vi "Evaluate Calibration.vi"(6 "Calibration Type":string, 7 "Position":u32, 8 "Error in":errorcluster caption="Error in (no error)", 9 "DSPic Measurement":dbl, 10 "Actual Measurement":dbl, 11 "Calibration in":refnum<class "Calibration.lvclass">) -> (0 "Error out":errorcluster, 3 "Passed":bool)   [LabVIEW 2015, in "Calibration.lvclass"]
uses:
  Calibration.lvclass
  <vilib>/Cree, Inc/Cree Test Framework/Core Launcher/Core Manager Methods -- Enum.ctl
  CBTF Applications/Driver Board Testing/Main/Application/Application/Class/Driver Board Test.lvclass
  <vilib>/Cree, Inc/Cree Test Framework/Core Launcher/Core Launcher.lvlib
  <vilib>/Cree, Inc/Cree Test Framework/Classes/Data/Data Repo/Class/Data Repo.lvclass
  Test Class/Test Class.lvclass
  Classes/Application/Class/Application.lvclass
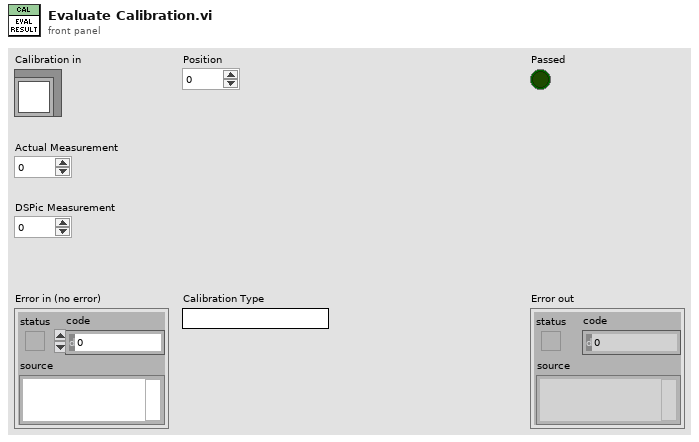
[diagram p1: front panel]
types:
  T1 = typedef "Core Launcher.lvlib/Core Manager Methods -- Enum.ctl" = enum16{"Spawn Objects", "Get Objects", "Destroy Objects"}
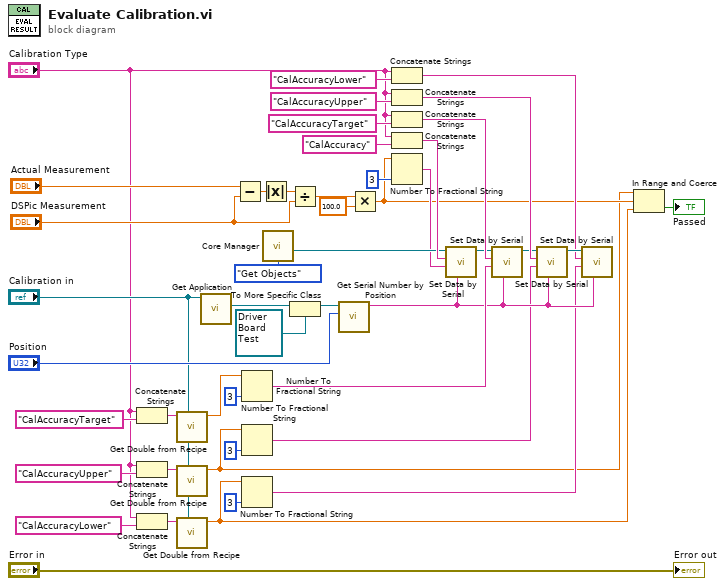
[diagram p0: block diagram]
diagram:
  n1 = Concatenate Strings("Calibration Type", "CalAccuracyTarget" ("Name")) -> (w26:string)
  n2 = Concatenate Strings("Calibration Type", "CalAccuracyUpper" ("string")) -> (w14:string)
  n3 = Concatenate Strings("Calibration Type", "CalAccuracyLower" ("string")) -> (w16:string)
  n4 = call "Get Double from Recipe.vi"("Test Class in"="Calibration in", "Name"=w26) -> ("Value"=w24:dbl)  [unwired: 7 in, 2 out]
  n5 = call "Get Double from Recipe.vi"("Test Class in"="Calibration in", "Name"=w14) -> ("Value"=w4:dbl)  [unwired: 7 in, 2 out]
  n6 = call "Get Double from Recipe.vi"("Test Class in"="Calibration in", "Name"=w16) -> ("Value"=w5:dbl)  [unwired: 7 in, 2 out]
  n7 = call "Get Application.vi"("Test Class in"="Calibration in") -> ("Application.lvlib:Application.lvclass"=w32:refnum<class "Application.lvclass">)  [unwired: 9 in, 1 out]
  n8 = Subtract(x="Actual Measurement", y="DSPic Measurement") -> (x-y=w45:dbl)
  n9 = Number To Fractional String(number=w24, precision (6)=i16 3 ("width (-)")) -> (F-format string=w23:string)  [unwired: 2 in]
  n10 = Number To Fractional String(number=w4, precision (6)=i16 3 ("width (-)")) -> (F-format string=w8:string)  [unwired: 2 in]
  n11 = Number To Fractional String(number=w5, precision (6)=i16 3 ("width (-)")) -> (F-format string=w7:string)  [unwired: 2 in]
  n12 = Absolute Value(x=w45) -> (abs(x)=w41:dbl)
  n13 = call <vilib>:"Core Manager.vi"("Method"=Core_Manager_Methods_--_Enum."Get Objects") -> ("Data Repo"=w36:refnum<class "Data Repo.lvclass">)  [unwired: 6 in, 4 out]
  n14 = Divide(x=w41, y="DSPic Measurement") -> (x/y=w43:dbl)
  n15 = To More Specific Class(target class=refnum<class "Driver Board Test.lvclass"> refnum ("Driver Board Test in"), reference=w32) -> (specific class reference=w34:refnum<class "Driver Board Test.lvclass">)  [unwired: 1 in, 1 out]
  n16 = call "Get Serial Number by Position.vi"("Position"="Position", "Application.lvclass"=w34) -> ("Value"=w11:string)  [unwired: 9 in]
  n17 = Multiply(x=w43, y=100.0) -> (x*y=w6:dbl)
  n18 = Concatenate Strings("Calibration Type", "CalAccuracyLower" ("string")) -> (w9:string)
  n19 = Concatenate Strings("Calibration Type", "CalAccuracyUpper" ("string")) -> (w13:string)
  n20 = Concatenate Strings("Calibration Type", "CalAccuracyTarget" ("string")) -> (w40:string)
  n21 = Concatenate Strings("Calibration Type", "CalAccuracy" ("string")) -> (w39:string)
  n22 = Number To Fractional String(number=w6, precision (6)=i16 3 ("width (-)")) -> (F-format string=w28:string)  [unwired: 2 in]
  n23 = call <vilib>:"Set Data by Serial.vi"("Serial"=w11, "Value"=w28, "Header"=w39, "Acrobat Template in"=w36) -> ("Acrobat Template out"=w35:refnum<class "Data Repo.lvclass">)  [unwired: 6 in, 1 out]
  n24 = call <vilib>:"Set Data by Serial.vi"("Serial"=w11, "Value"=w23, "Header"=w40, "Acrobat Template in"=w35) -> ("Acrobat Template out"=w12:refnum<class "Data Repo.lvclass">)  [unwired: 6 in, 1 out]
  n25 = call <vilib>:"Set Data by Serial.vi"("Serial"=w11, "Value"=w8, "Header"=w13, "Acrobat Template in"=w12) -> ("Acrobat Template out"=w10:refnum<class "Data Repo.lvclass">)  [unwired: 6 in, 1 out]
  n26 = call <vilib>:"Set Data by Serial.vi"("Serial"=w11, "Value"=w7, "Header"=w9, "Acrobat Template in"=w10) -> ()  [unwired: 6 in, 2 out]
  n27 = In Range and Coerce(upper limit=w4, x=w6, lower limit=w5) -> (In Range?=→"Passed":bool)  [unwired: 1 out]
  "Error out" <- "Error in"
